vi "Init.vi"(7 "I2C #":T1=-1, 8 "error in (no error)":errorcluster, 10 "Session In":refnum<class "Session.lvclass">) -> (0 "error out":errorcluster, 3 "Grove I2C L298P Motor Drive Out":refnum<class "Grove I2C L298P Motor Drive.lvclass">)   [LabVIEW 2020, in "CTI-Peripheral.lvlib" / "Grove I2C L298P Motor Drive.lvclass"]
uses:
  Grove I2C L298P Motor Drive.lvclass
  CTI/Session/Session.lvclass
  CTI/I2C Number.ctl
  CTI/I2C Address.ctl
  CTI/I2C Connection/I2C Connection.lvclass/I2C Connection.ctl
  Grove I2C L298P Motor Drive.lvclass/Grove I2C L298P Motor Drive.ctl
  CTI/I2C Connection/I2C Connection.lvclass
  CTI/CTI.lvlib
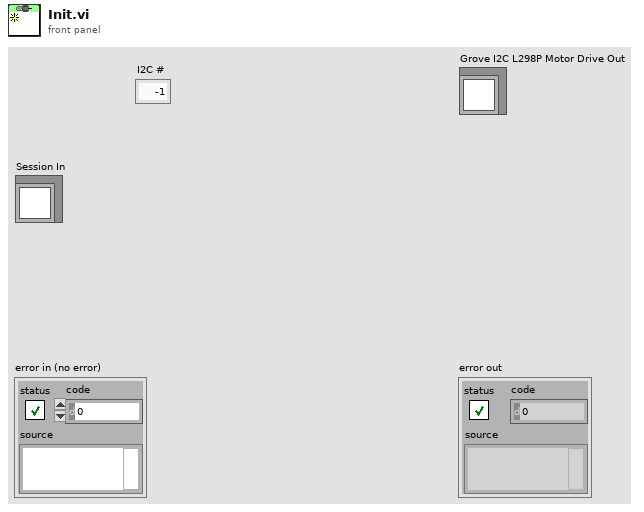
[diagram p1: front panel]
types:
  T1 = typedef "CTI.lvlib/I2C Number.ctl" = i8
  T2 = typedef "CTI.lvlib/I2C Address.ctl" = u8
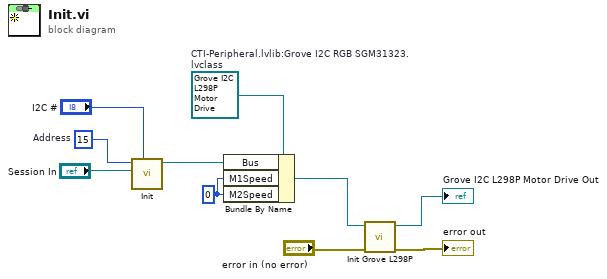
[diagram p0: block diagram]
diagram:
  w1 = u8 0 ("M2Speed")
  w6 = refnum<class "Grove I2C L298P Motor Drive.lvclass"> refnum  # CTI-Peripheral.lvlib:Grove I2C RGB SGM31323.lvclass
  w7 = T2 15  # Address
  n1 = call "Init.vi"("I2C #"="I2C #", "Session"="Session In", "Address"=w7) -> ("I2C Connection"=w10:refnum<class "I2C Connection.lvclass">)  [unwired: 7 in, 1 out]
  n2 = Bundle By Name(cluster=w6, "Bus"=w10, "M1Speed"=w1, "M2Speed"=w1) -> (w3:refnum<class "Grove I2C L298P Motor Drive.lvclass">)
  n3 = call "Init Grove L298P.vi"("error in (no error)"="error in (no error)", "Grove I2C L298P Motor Drive in"=w3) -> ("error out"=→"error out":errorcluster, "Grove I2C L298P Motor Drive out"=→"Grove I2C L298P Motor Drive Out":refnum<class "Grove I2C L298P Motor Drive.lvclass">)  [unwired: 8 in]
